vi "Add Always Included.vi"(8 "error in (no error)":errorcluster, 10 "ProjectItem Refnum":refnum<vi>, 11 "NI_AB_API_RESTful in":refnum<class "NI_AB_API_RESTful.lvclass">) -> (0 "error out":errorcluster, 3 "NI_AB_API_RESTful out":refnum<class "NI_AB_API_RESTful.lvclass">)   [LabVIEW 2020, in "NI_AB_API_RESTful.lvclass"]
uses:
  <vilib>/AppBuilder/AB_API/RESTful/NI_AB_API_RESTful.lvclass
  <vilib>/AppBuilder/AB_API/RESTful/NI_AB_API_RESTful.lvclass/NI_AB_API_RESTful.ctl
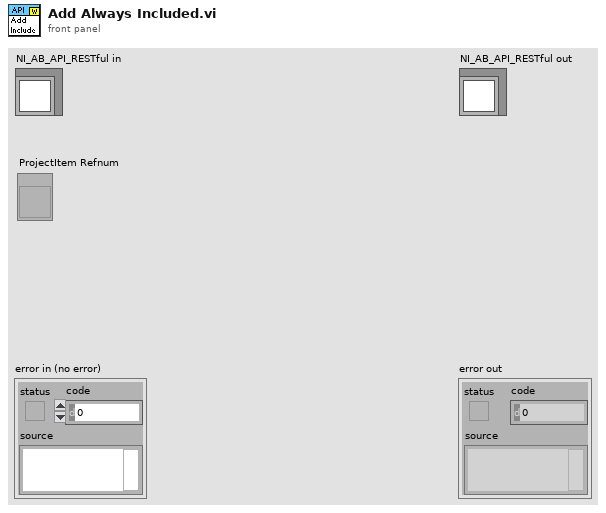
[diagram p1: front panel]
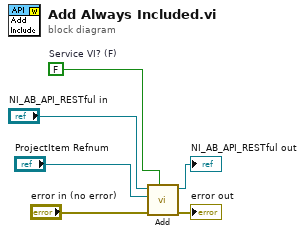
[diagram p0: block diagram]
diagram:
  w2 = FALSE  # Service VI? (F)
  n1 = call <vilib>:"Add.vi"("Service VI? (F)"=w2, "error in (no error)"="error in (no error)", "ProjectItem Refnum"="ProjectItem Refnum", "NI_AB_API_RESTful in"="NI_AB_API_RESTful in") -> ("error out"=→"error out":errorcluster, "NI_AB_API_RESTful out"=→"NI_AB_API_RESTful out":refnum<class "NI_AB_API_RESTful.lvclass">)  [unwired: 6 in]
